vi "Block Profile Measurement.vi"() -> ()   [LabVIEW 2011]
uses:
  <vilib>/DAQmx/read.llb/DAQmx Read (Analog Wfm 1Chan NSamp).vi
  <vilib>/DAQmx/create/channels.llb/DAQmx Create Channel (AI-Current-Basic).vi
  <vilib>/DAQmx/configure/timing.llb/DAQmx Timing (Sample Clock).vi
  <vilib>/DAQmx/miscellaneous.llb/DAQmx Fill In Error Info.vi
  <vilib>/Analysis/NI_AALBase.lvlib
panel:
  in  "ECOLAB Button":bool
  out "Max Value":dbl
  out "Maximum":string
  out "Block Count":i32
  in  "Tab Control":enum32{"DISPLAY", "CONFIG", "CALIBRATE"}(tab)
  in  "Intervals":i32=20
  in  "Rate (Inches / Second)":dbl=12.0
  out "XY Graph":cluster{dbl[], "Initialize Value":dbl[]}(graph)
  out "Histogram Graph":T1(graph)
  out "Save Error":errorcluster
  out "Distance Between Measurements (Inches)":dbl=0.024
  out "dt":dbl=0.002
  out "Main Error":errorcluster
  out "DAQ Error":errorcluster
  in  "DAQ Selection":tag="cDAQ1Mod1/ai0"
  in  "Samples/Channel":i32=5
  in  "Sample Rate (Hz)":dbl=500.0
  in  "Comments (Saves to Data File)":string
  out "DAQ Loop":i32=1303
  out "File Path Output":path=path "H:/Projects/Chris Opelt/Data Files/Data-12-22-2011-{3-PM}.xls"
  in  "Scale Template":T2={"Channel Select"=0, "Clear/Reset Scales"=FALSE, "Channel #"=["0"], "Scale Names"=["0"], "Set?"=[FALSE, FALSE], "HI/LO Setpoints"=[1.0, 0.0], "Units"=["0"], "HI/LO Signals"=[1.0, 0.0], "Slope/Intercept"=[1.0, 0.0], "IN/OUT Values"=[0.0038010106989999994, 0.0038010106989999994]} {"Channel Select" min=0 step=1; "Slope/Intercept" format="%#.3p"; "HI/LO Setpoints" format="%#.3p"; "IN/OUT Values" format="%.3p"; "HI/LO Signals" format="%#.3p"}
  in  "Simulate Signal?":bool
  in  "Simulated Signal":dbl
  in  "Stop Program":bool=TRUE
  in  "Analyze Data?":bool
  in  "Reset Block Count?":bool
  in  "Distance Threshold (> = Measure)":dbl=0.004
  in  "Save Data Signal":bool
  # "Threshold (inches)"
  # "Block Count"
  # "Maximum (inches)"
  # "Block Profile Measurement Program"
  # "Blake Otting - 2011"
  # "Histogram of Maximum Value Measurements"
  # "Measurement Profile of Last Block"
  # "Track Rate"
  # "Inches / Second"
  # "Ch.\n#"
  # "Scale\nName"
  # "Set\nValues?"
  # "Scaled"
  # "Pre-Scaled"
  # "Scaling Result"
  # "Values"
  # "Units"
  # "Values"
  # "Channel\nSelect"
  # "HI"
  # "Slope"
  # "IN"
  # "LO"
  # "Intercept"
  # "OUT"
  # "HI"
  # "Slope"
  # "IN"
  # "LO"
  # "Intercept"
  # "OUT"
  # "HI"
  # "Slope"
  # "IN"
  # "LO"
  # "Intercept"
  # "OUT"
  # "HI"
  # "Slope"
  # "IN"
  # "LO"
  # "Intercept"
  # "OUT"
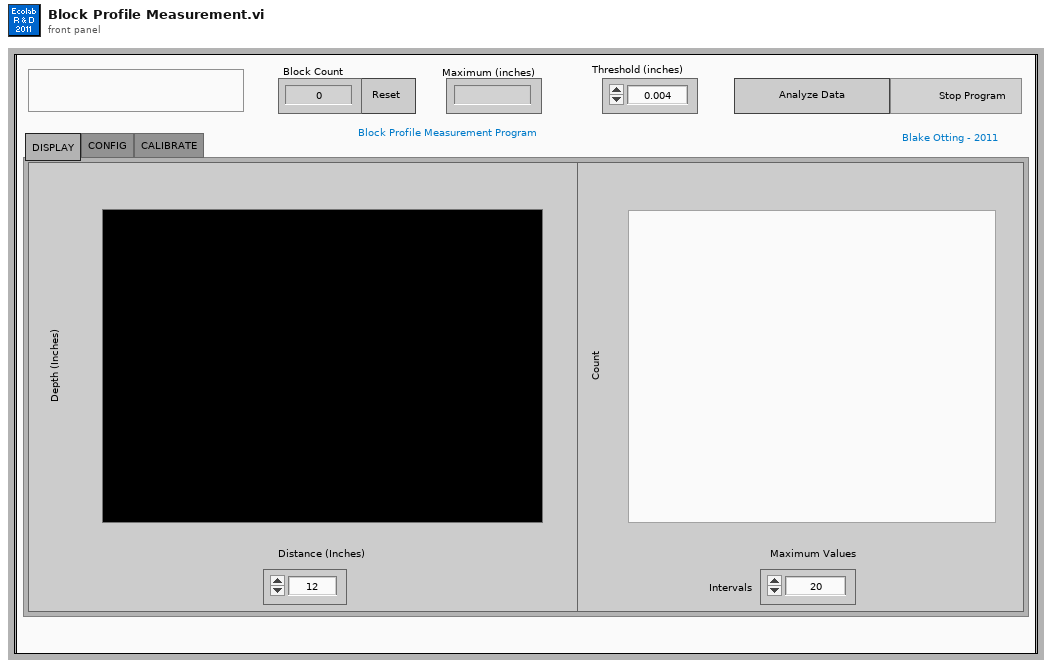
[diagram p1: front panel]
types:
  T1 = cluster{"X Values":dbl[], "Histogram: h(x)":i32[]}
  T2 = cluster{"Channel Select":i32, "Clear/Reset Scales":bool, "Channel #":string[], "Scale Names":string[], "Set?":bool[], "HI/LO Setpoints":dbl[], "Units":string[], "HI/LO Signals":dbl[], "Slope/Intercept":dbl[], "IN/OUT Values":dbl[]}
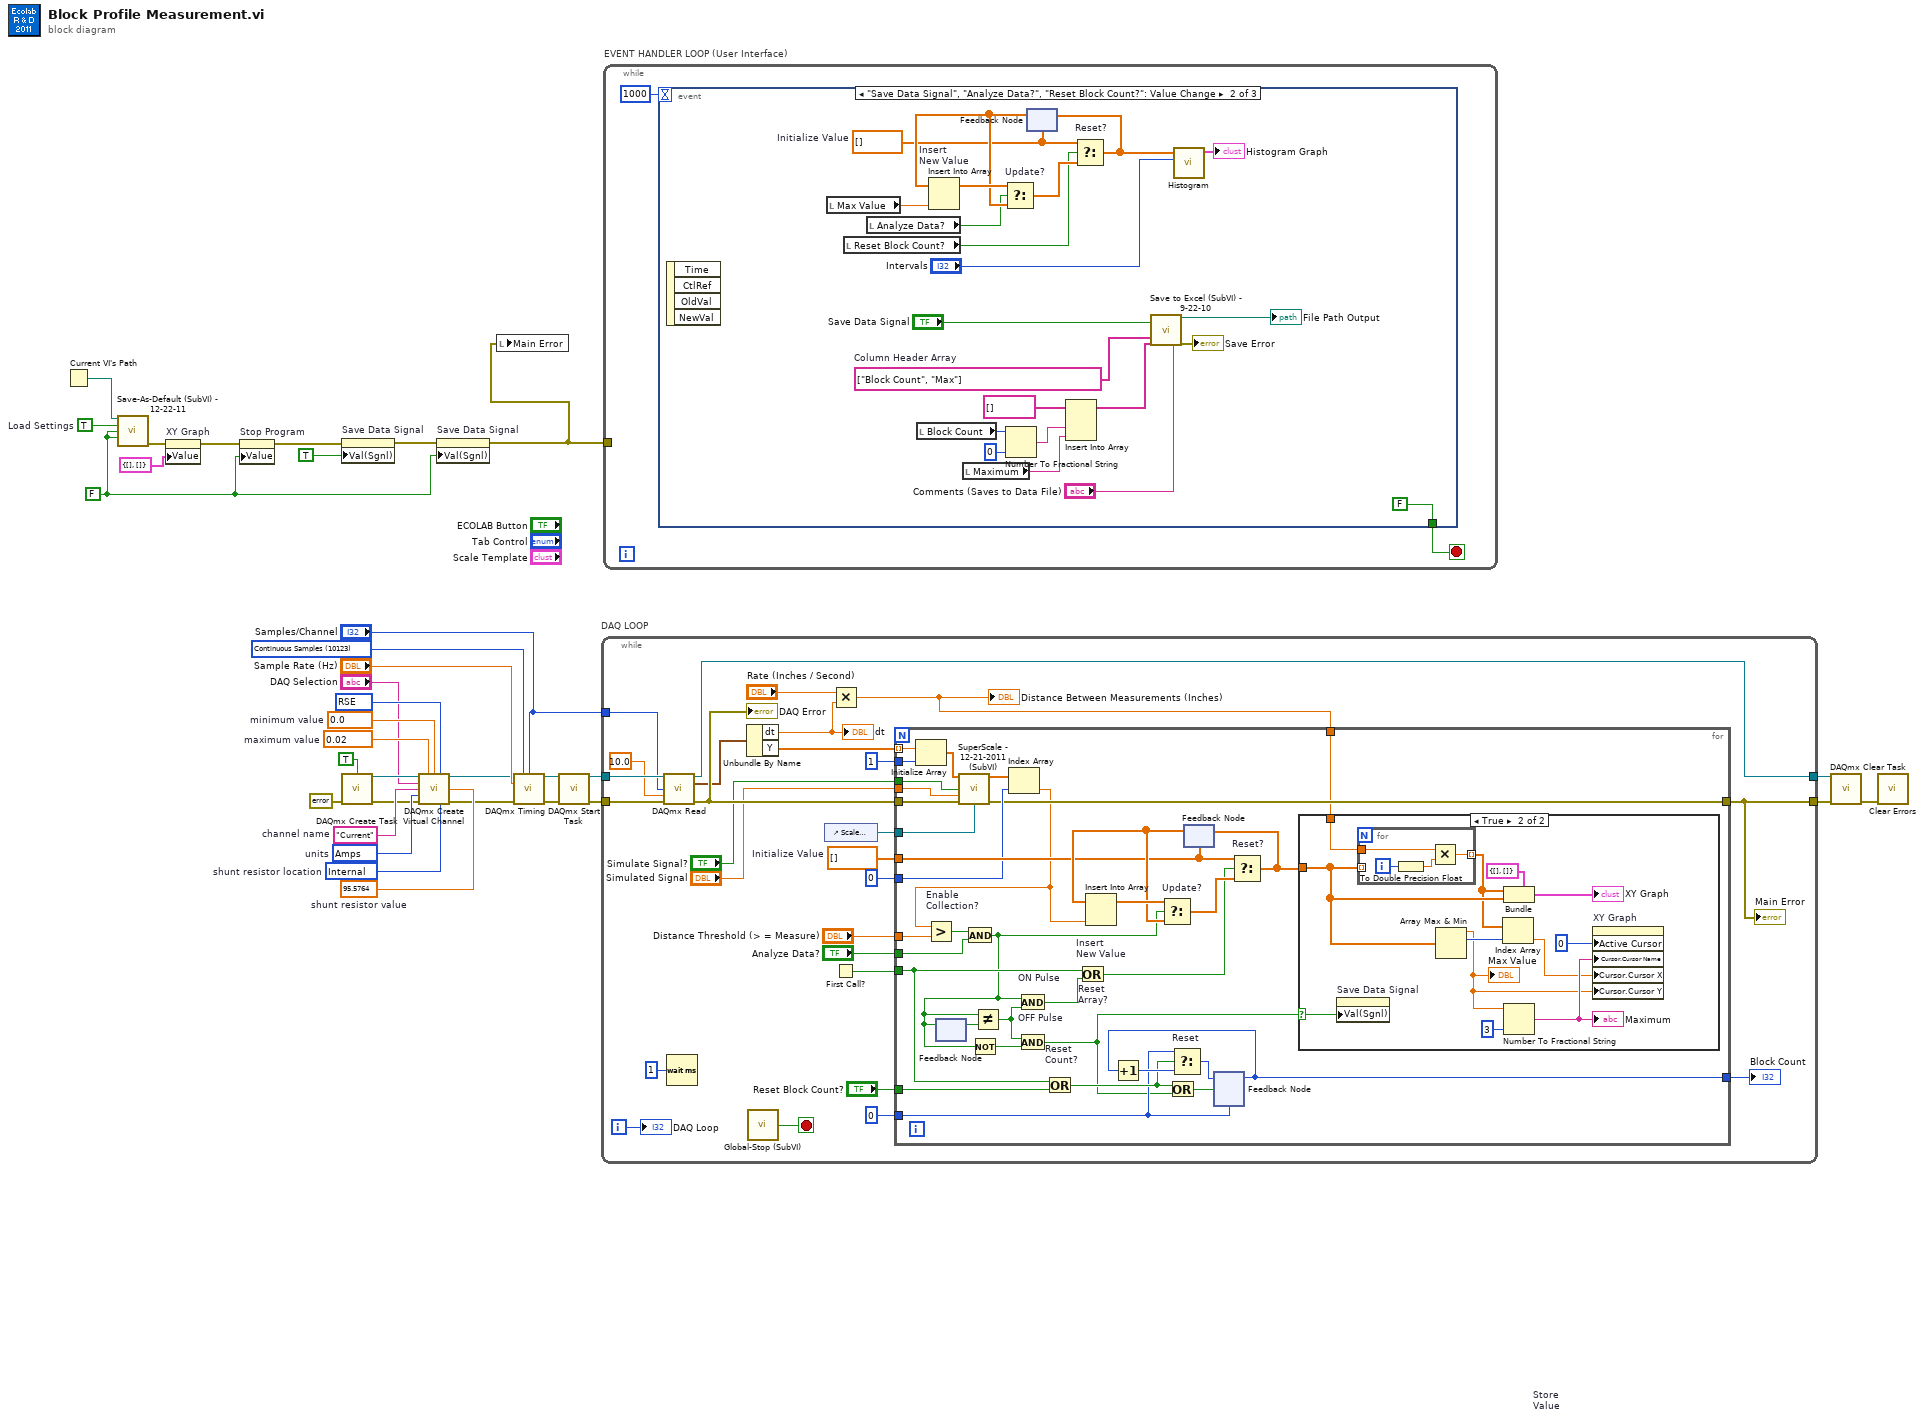
[diagram p0: block diagram]
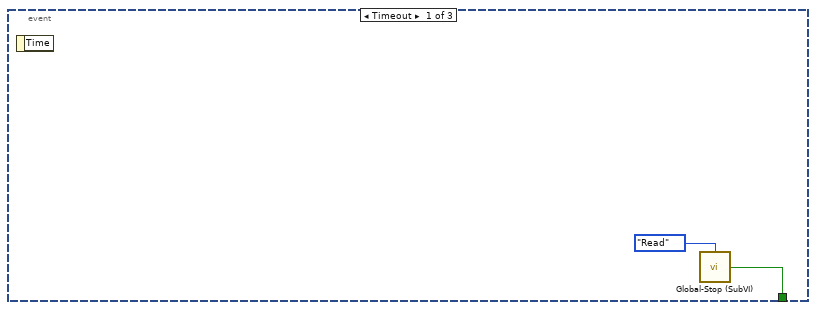
[diagram p2: hidden frame]
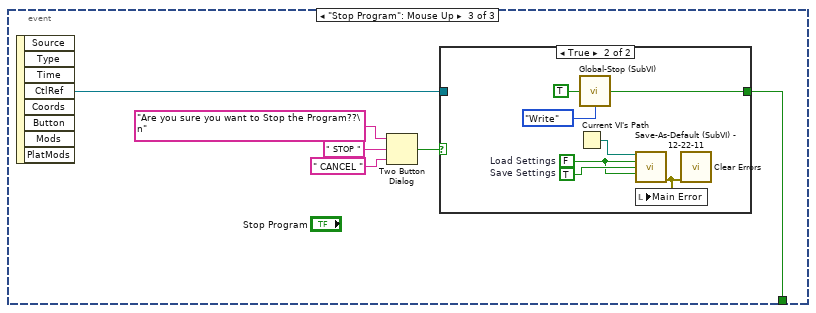
[diagram p3: hidden frame]
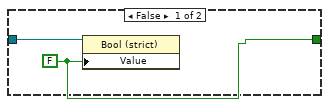
[diagram p4: hidden frame]
diagram:
  w6 = TRUE  # Load Settings
  w5 = FALSE
  w18 = 10123 items=["Finite Samples"=10178, "Continuous Samples"=10123, "Hardware Timed Single Point"=12522] ("Sample Mode")
  w26 = 10083 items=["default"=-1, "RSE"=10083, "NRSE"=10078, "Differential"=10106, "Pseudodifferential"=12529]
  w27 = 10342 items=["Amps"=10342, "From Custom Scale"=10065]  # units
  w28 = 95.5764  # shunt resistor value
  w29 = 10200 items=["Internal"=10200, "External"=10167]  # shunt resistor location
  w30 = "Current"  # channel name
  w31 = 0.0  # minimum value
  w32 = 0.02  # maximum value
  n1 = Current VI's Path() -> (path=w7:path)
  n2 = call "Save-As-Default (SubVI) - 12-22-11.vi"("Current VI's Path"=w7, "Load Settings"=w6, "Save Settings"=w5, "Save and Exit"=w5) -> ("Error Output"=w4:errorcluster)  [unwired: 11 in]
  n3 = property on="XY Graph" class="XYGraph (strict)"(error in=w4, "Value"=cluster{dbl[], "Initialize Value":dbl[]} {[], "Initialize Value"=[]} ("XY Graph")) -> (error out=w3:errorcluster)  [unwired: 1 in, 1 out]
  n4 = property on="Stop Program" class="Bool (strict)"(error in=w3, "Value"=w5) -> (error out=w8:errorcluster)  [unwired: 1 in, 1 out]
  n5 = property on="Save Data Signal" class="Bool (strict)"(error in=w8, "Val(Sgnl)"=TRUE) -> (error out=w9:errorcluster)  [unwired: 1 in, 1 out]
  n6 = call <vilib>:"DAQmx Create Task.vi"("auto cleanup"=TRUE, "error in"=errorcluster {"status"=FALSE, "code"=0, "source"=""}) -> ("task out"=w25:refnum<k21>, "error out"=w24:errorcluster)  [unwired: 12 in]
  n7 = call-poly <vilib>:"DAQmx Create Virtual Channel.vi"("task in"=w25, "maximum value"=w32, "minimum value"=w31, "input terminal configuration"=w26, "physical channels"="DAQ Selection", "name to assign"=w30, "external shunt resistor value"=w28, "units"=w27, "error in"=w24, "shunt resistor location"=w29) -> ("task out"=w17:refnum<k21>, "error out"=w16:errorcluster)  [unwired: 1 in, 3 out]
  n8 = property on="Save Data Signal" class="Bool (strict)"(error in=w9, "Val(Sgnl)"=w5) -> (error out=w1:errorcluster)  [unwired: 1 in, 1 out]
  n9 = local write "Main Error"(w1) -> ()
  n10 = call-poly <vilib>:"DAQmx Timing.vi"("task/channels in"=w17, "sample mode"=w18, "samples per channel"="Samples/Channel", "rate"="Sample Rate (Hz)", "error in"=w16) -> ("task out"=w14:refnum<k21>, "error out"=w15:errorcluster)  [unwired: 2 in, 7 out]
  n11 = call <vilib>:"DAQmx Start Task.vi"("task/channels in"=w14, "error in"=w15) -> ("task out"=w13:refnum<k21>, "error out"=w12:errorcluster)  [unwired: 12 in]
  n12 = while "DAQ LOOP" {
    tunnel: [w35] -> w33
    tunnel: w12 -> [w48]
    tunnel: w13 -> [w49]
    tunnel: [w39] -> w20
    tunnel: "Samples/Channel" -> [w47]
    i -> [w61]
    stop <- w40 stop-if-true
    w50 = dbl[] []  # Initialize Value
    n13 = call-poly <vilib>:"DAQmx Read.vi"("task/channels in"=w49, "number of samples per channel"=w47, "timeout"=10.0, "error in"=w48) -> ("task out"=w35:refnum<k21>, "data"=w44:waveform(dbl), "error out"=w45:errorcluster)  [unwired: 9 in]
    "DAQ Error" <- w45
    n14 = Wait (ms)(milliseconds to wait=u32 1) -> ()  [unwired: 1 out]
    n15 = Unbundle By Name(w44) -> ("dt"=w42:dbl, "Y"=w43:dbl[])
    "dt" <- w42
    n16 = call "Global-Stop (SubVI).vi"() -> ("OUT"=w40:bool)  [unwired: 4 in]
    n17 = control-ref of="Scale Template"() -> (w55:refnum<vi>)
    n18 = Multiply(x="Rate (Inches / Second)", y=w42) -> (x*y=w36:dbl)
    "Distance Between Measurements (Inches)" <- w36
    n19 = First Call?() -> (First Call?: T/F=w54:bool)
    n20 = for {
      tunnel: w43 -> [w96] mode=indexing
      tunnel: "Distance Threshold (> = Measure)" -> [w65]
      tunnel: "Analyze Data?" -> [w80]
      tunnel: w50 -> [w79]
      tunnel: 1 ("dimension size") -> [w77]
      tunnel: 0 ("index") -> [w76]
      tunnel: 0 ("index") -> [w75]
      tunnel: w54 -> [w74]
      tunnel: "Reset Block Count?" -> [w73]
      tunnel: [w72] -> w39
      tunnel: w45 -> [w71]
      tunnel: w55 -> [w70]
      tunnel: [w67] -> w56
      tunnel: w36 -> [w68]
      tunnel: "Simulate Signal?" -> [w64]
      tunnel: "Simulated Signal" -> [w63]
      n21 = Initialize Array(w96, w77) -> (w95:dbl[])
      n22 = feedback #1() -> (w88:bool)  [unwired: 1 in]
      n23 = call "SuperScale - 12-21-2011 (SubVI).vi"("Measured Signals"=w95, "Simulate Signal?"=w64, "Simulated Signal"=w63, "Error Input"=w71, "Scale Ref"=w70) -> ("Scaled Values"=w94:dbl[], "Scale Error"=w72:errorcluster)  [unwired: 9 in]
      n24 = Index Array(array=w94, index=w76) -> (element=w69:dbl)
      n25 = Greater? "Enable\nCollection?"(x=w69, y=w65) -> (0:w93:bool)
      n26 = And(x=w93, y=w80) -> (x .and. y?=w62:bool)
      n27 = feedback-in #1(w62) -> ()
      n28 = Not(x=w62) -> (.not. x?=w86:bool)
      n29 = Not Equal?(x=w62, y=w88) -> (x != y?=w87:bool)
      n30 = And "ON Pulse"(x=w62, y=w87) -> (x .and. y?=w82:bool)
      n31 = And "OFF Pulse"(x=w87, y=w86) -> (x .and. y?=w66:bool)
      n32 = Or "Reset\nCount?"(x=w74, y=w73) -> (x .or. y?=w81:bool)
      n33 = Or "Reset\nArray?"(x=w74, y=w82) -> (x .or. y?=w89:bool)
      n34 = Or(x=w81, y=w66) -> (x .or. y?=w83:bool)
      n35 = feedback #2(w79) -> (w91:dbl[])
      n36 = Insert Into Array "Insert \nNew Value"(array=w91, new element=w69) -> (w92:dbl[])  [unwired: 1 in]
      n37 = Select "Update?"(t=w92, s=w62, f=w91) -> (s? t:f=w90:dbl[])
      n38 = feedback #3 "Store\nValue"(w75) -> (w67:i32)
      n39 = Increment(x=w67) -> (x+1=w85:i32)
      n40 = Select "Reset"(t=w75, s=w81, f=w85) -> (s? t:f=w84:i32)
      n41 = feedback-in #3(w84, w83) -> ()
      n42 = Select "Reset?"(t=w79, s=w89, f=w90) -> (s? t:f=w78:dbl[])
      n43 = feedback-in #2(w78) -> ()
      n44 = case shown="True" w66 {
        selector: w66 -> [_ w97]
        tunnel: w78 -> [_ w107]
        tunnel: w68 -> [_ w108]
        frame False {
        }
        frame True {
          n45 = property on="Save Data Signal" class="Bool (strict)"("Val(Sgnl)"=w97) -> ()  [unwired: 2 in, 2 out]
          n46 = for {
            tunnel: w107 -> [_] mode=indexing
            tunnel: w108 -> [w112]
            tunnel: [w109] -> w105 mode=indexing
            i -> [w110]
            n47 = To Double Precision Float(number=w110) -> (double precision float=w111:dbl)
            n48 = Multiply(x=w112, y=w111) -> (x*y=w109:dbl)
          }
          n49 = Array Max & Min(array=w107) -> (max value=w99:dbl, max index (indices)=w104:i32)  [unwired: 2 out]
          "Max Value" <- w99
          n50 = Index Array(array=w105, index=w104) -> (element=w100:dbl)
          n51 = Bundle(cluster=cluster{dbl[], "Initialize Value":dbl[]} {[], "Initialize Value"=[]}, w105, "Initialize Value"=w107) -> (→"XY Graph":cluster{dbl[], "Initialize Value":dbl[]})
          n52 = Number To Fractional String(number=w99, precision (6)=i16 3) -> (F-format string=w101:string)  [unwired: 2 in]
          "Maximum" <- w101
          n53 = property on="XY Graph" class="XYGraph (strict)"("Active Cursor"=u32 0, "Cursor.Cursor Name"=w101, "Cursor.Cursor X"=w100, "Cursor.Cursor Y"=w99) -> ()  [unwired: 2 in, 2 out]
        }
      }
    }
    "Block Count" <- w56
    "Main Error" <- w39
    "DAQ Loop" <- w61
  }
  n54 = while "EVENT HANDLER LOOP (User Interface)" {
    tunnel: w1 -> [_]
    stop <- w114 stop-if-true
    n55 = event shown="[1] \"Save Data Signal\", \"Analyze Data?\", \"Reset Block Count?\": Value Change" {
      selector: _ -> [_ _ _]
      dyn-events: _ -> [_ _ _]
      timeout: 1000 -> [_ _ _]
      tunnel: [w115 FALSE ("OUT") w140] -> w114
      event Timeout {
        n56 = event-data() -> ()  [unwired: 2 out]
        n57 = call "Global-Stop (SubVI).vi"("Mode (Read)"=enum16{"Read", "Write"}."Read") -> ("OUT"=w115:bool)  [unwired: 3 in]
      }
      event "Save Data Signal", "Analyze Data?", "Reset Block Count?": Value Change {
        w122 = string[] ["Block Count", "Max"]  # Column Header Array
        w134 = dbl[] []  # Initialize Value
        n58 = event-data() -> ()  [unwired: 5 out]
        n59 = local read "Max Value"() -> (w131:dbl)
        n60 = local read "Reset Block Count?"() -> (w133:bool)
        n61 = local read "Analyze Data?"() -> (w132:bool)
        n62 = local read "Block Count"() -> (w126:i32)
        n63 = local read "Maximum"() -> (w119:string)
        n64 = Number To Fractional String(number=w126, precision (6)=i16 0) -> (F-format string=w127:string)  [unwired: 2 in]
        n65 = feedback #4(w134) -> (w136:dbl[])
        n66 = Insert Into Array "Insert \nNew Value"(array=w136, new element=w131) -> (w137:dbl[])  [unwired: 1 in]
        n67 = Select "Update?"(t=w137, s=w132, f=w136) -> (s? t:f=w135:dbl[])
        n68 = Insert Into Array(array=string[] [] ("F-format string"), new element #1=w127, new element #2=w119) -> (w123:string[])  [unwired: 1 in]
        n69 = Select "Reset?"(t=w134, s=w133, f=w135) -> (s? t:f=w130:dbl[])
        n70 = feedback-in #4(w130) -> ()
        n71 = call "Save to Excel (SubVI) - 9-22-10.vi"("Save (Enable/Signal)"="Save Data Signal", "Column Header Array"=w122, "Data Array (Row)"=w123, "Comments"="Comments (Saves to Data File)") -> ("File Path Output"=→"File Path Output":path, "Error Output"=→"Save Error":errorcluster)  [unwired: 11 in, 3 out]
        n72 = call <vilib>:"Histogram.vi"("intervals"="Intervals", "X"=w130) -> ("Histogram Graph"=→"Histogram Graph":T1)  [unwired: 6 in, 3 out]
      }
      event "Stop Program": Mouse Up {
        n73 = event-data() -> ("CtlRef"=w139:refnum<vi>)  [unwired: 8 out]
        n74 = Two Button Dialog(message="Are you sure you want to Stop the Program??\n", 1:" CANCEL " ("F button name (\"Cancel\")"), 2:" STOP ") -> (T button?=w141:bool)
        n75 = case shown="True" w141 {
          tunnel: [w145 w151] -> w140
          tunnel: w139 -> [w146 _]
          frame False {
            w145 = FALSE ("Value")
            n76 = property class="Bool (strict)"(reference=w146, "Value"=w145) -> ()  [unwired: 1 in, 2 out]
          }
          frame True {
            w149 = TRUE  # Save Settings
            w148 = FALSE  # Load Settings
            n77 = Current VI's Path() -> (path=w150:path)
            n78 = call "Global-Stop (SubVI).vi"("Mode (Read)"=enum16{"Read", "Write"}."Write", "IN"=TRUE) -> ("OUT"=w151:bool)  [unwired: 2 in]
            n79 = call "Save-As-Default (SubVI) - 12-22-11.vi"("Current VI's Path"=w150, "Load Settings"=w148, "Save Settings"=w149, "Save and Exit"=w148) -> ("Error Output"=w147:errorcluster)  [unwired: 11 in]
            n80 = local write "Main Error"(w147) -> ()
            n81 = call <vilib>:"Clear Errors.vi"("error in (no error)"=w147) -> ()  [unwired: 7 out]
          }
        }
      }
    }
  }
  n82 = call <vilib>:"DAQmx Clear Task.vi"("task in"=w33, "error in"=w20) -> ("error out"=w34:errorcluster)  [unwired: 13 out]
  n83 = call <vilib>:"Clear Errors.vi"("error in (no error)"=w34) -> ()  [unwired: 6 in, 1 out]
